vi "ZCAN_SEND.vi"(5 "CANFD_SpeedUp":u32, 6 "Data":string="11 22 33 44 55 66 77 88", 7 "ID":u32=18 format="0x%08x", 8 "error IO":errorcluster, 9 "agreement":T1, 10 "frame type":T2, 11 "can_index_handle":u32) -> (0 "error out":errorcluster)   [LabVIEW 2020, in "zlgcan.lvlib"]
uses:
  zlgcan.lvlib
  data_type/frame type.ctl
  data_type/Agreement.ctl
  data_type/ZCAN_TransmitFD_Data.ctl
  data_type/ZCAN_Transmit_Data.ctl
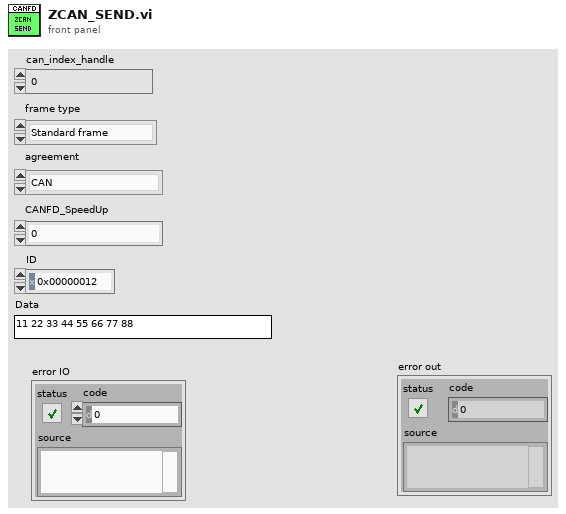
[diagram p1: front panel]
types:
  T1 = typedef "zlgcan.lvlib/Agreement.ctl" = enum16{"CAN", "CANFD"}
  T2 = typedef "zlgcan.lvlib/frame type.ctl" = enum32{"Standard frame", "Extended frame"}
  T3 = typedef "zlgcan.lvlib/ZCAN_TransmitFD_Data.ctl" = cluster{"帧类型":u32, "帧格式":u32, "ID":u32, "数据长度":u8, "CANFD加速？":u8, "DATA":cluster{"CAN数据[0]":u8, "CAN数据[1]":u8, "CAN数据[2]":u8, "CAN数据[3]":u8, "CAN数据[4]":u8, "CAN数据[5]":u8, "CAN数据[6]":u8, "CAN数据[7]":u8, "CAN数据[8]":u8, "CAN数据[9]":u8, "CAN数据[10]":u8, "CAN数据[11] ":u8, "CAN数据[12] ":u8, "CAN数据[13] ":u8, "CAN数据[14] ":u8, "CAN数据[15] ":u8, "CAN数据[16]":u8, "CAN数据[17]":u8, "CAN数据[18]":u8, "CAN数据[19]":u8, "CAN数据[20]":u8, "CAN数据[21]":u8, "CAN数据[22]":u8, "CAN数据[23]":u8, "CAN数据[24] ":u8, "CAN数据[25]":u8, "CAN数据[26]":u8, "CAN数据[27]":u8, "CAN数据[28]":u8, "CAN数据[29]":u8, "CAN数据[30]":u8, "CAN数据[31]":u8, "CAN数据[32]":u8, "CAN数据[33]":u8, "CAN数据[34]":u8, "CAN数据[35]":u8, "CAN数据[36]":u8, "CAN数据[37]":u8, "CAN数据[38]":u8, "CAN数据[39]":u8, "CAN数据[40]":u8, "CAN数据[41]":u8, "CAN数据[42]":u8, "CAN数据[43]":u8, "CAN数据[44]":u8, "CAN数据[45]":u8, "CAN数据[46]":u8, "CAN数据[47]":u8, "CAN数据[48]":u8, "CAN数据[49]":u8, "CAN数据[50]":u8, "CAN数据[51]":u8, "CAN数据[52]":u8, "CAN数据[53]":u8, "CAN数据[54]":u8, "CAN数据[55]":u8, "CAN数据[56]":u8, "CAN数据[57]":u8, "CAN数据[58]":u8, "CAN数据[59]":u8, "CAN数据[60]":u8, "CAN数据[61]":u8, "CAN数据[62]":u8, "CAN数据[63]":u8}, "发送方式":u32}
  T4 = typedef "zlgcan.lvlib/ZCAN_Transmit_Data.ctl" = cluster{"帧类型":u32, "帧格式":u32, "ID":u32, "数据长度":u8, "DATA":cluster{"CAN数据[0]":u8, "CAN数据[1]":u8, "CAN数据[2]":u8, "CAN数据[3]":u8, "CAN数据[4]":u8, "CAN数据[5]":u8, "CAN数据[6]":u8, "CAN数据[7]":u8}, "发送方式":u32}
  T5 = cluster{"[0]":u32, "[1]":u32, "[2]":u32, "[3]":u32, "[4]":u32, "[5]":u32, "[6]":u32, "[7]":u32, "[8]":u32, "[9]":u32, "[10]":u32, "[11]":u32, "[12]":u32, "[13]":u32, "[14]":u32, "[15]":u32, "[16]":u32, "[17]":u32, "[18]":u32, "[19]":u32, "[20]":u32, "[21]":u32, "[22]":u32, "[23]":u32, "[24]":u32, "[25]":u32, "[26]":u32, "[27]":u32, "[28]":u32, "[29]":u32, "[30]":u32, "[31]":u32, "[32]":u32, "[33]":u32, "[34]":u32, "[35]":u32, "[36]":u32, "[37]":u32, "[38]":u32, "[39]":u32, "[40]":u32, "[41]":u32, "[42]":u32, "[43]":u32, "[44]":u32, "[45]":u32, "[46]":u32, "[47]":u32, "[48]":u32, "[49]":u32, "[50]":u32, "[51]":u32, "[52]":u32, "[53]":u32, "[54]":u32, "[55]":u32, "[56]":u32, "[57]":u32, "[58]":u32, "[59]":u32, "[60]":u32, "[61]":u32, "[62]":u32, "[63]":u32}
  T6 = cluster{"[0]":u32, "[1]":u32, "[2]":u32, "[3]":u32, "[4]":u32, "[5]":u32, "[6]":u32, "[7]":u32}
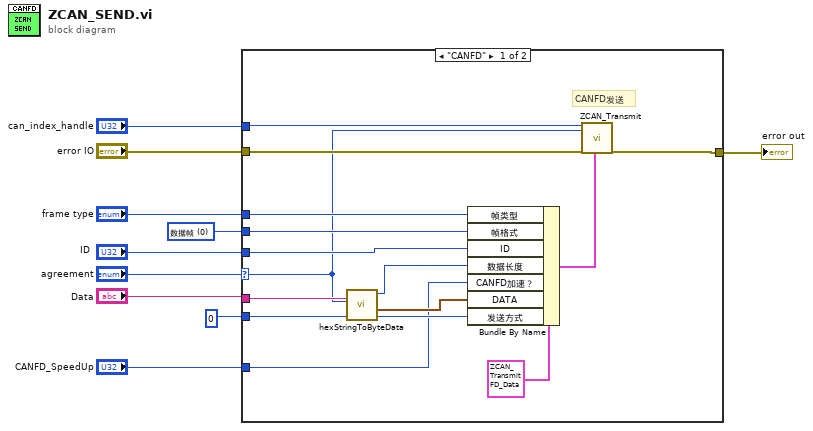
[diagram p0: block diagram]
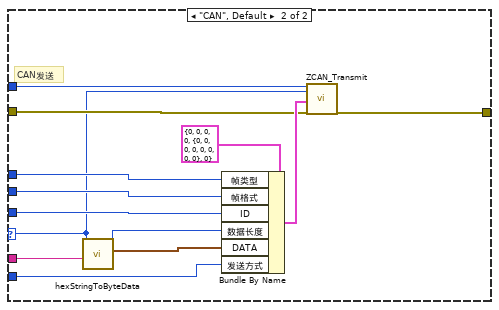
[diagram p2: hidden frame]
diagram:
  w8 = u32 0 items=["数据帧", "远程帧"] ("帧格式")
  n1 = case shown="\"CANFD\"" "agreement" {
    selector: "agreement" -> [w13 w26]
    tunnel: "frame type" -> [w23 w36]
    tunnel: w8 -> [w22 w35]
    tunnel: "ID" -> [w21 w34]
    tunnel: u32 0 ("Send Type") -> [w20 w32]
    tunnel: "Data" -> [w18 w30]
    tunnel: "error IO" -> [w16 w28]
    tunnel: "can_index_handle" -> [w14 w27]
    tunnel: [w12 w25] -> w3
    tunnel: "CANFD_SpeedUp" -> [w11 _]
    frame "CANFD" {
      # "CANFD发送"
      n2 = call "hexStringToByteData.vi"("数据输入"=w18, "协议"=w13) -> ("CANFD_data"=w19:T5, "字节数"=w17:i32)  [unwired: 7 in, 1 out]
      n3 = Bundle By Name(cluster=T3 {"帧类型"=0, "帧格式"=0, "ID"=0, "数据长度"=0, "CANFD加速？"=0, "DATA"={"CAN数据[0]"=0, "CAN数据[1]"=0, "CAN数据[2]"=0, "CAN数据[3]"=0, "CAN数据[4]"=0, "CAN数据[5]"=0, "CAN数据[6]"=0, "CAN数据[7]"=0, "CAN数据[8]"=0, "CAN数据[9]"=0, "CAN数据[10]"=0, "CAN数据[11] "=0, "CAN数据[12] "=0, "CAN数据[13] "=0, "CAN数据[14] "=0, "CAN数据[15] "=0, "CAN数据[16]"=0, "CAN数据[17]"=0, "CAN数据[18]"=0, "CAN数据[19]"=0, "CAN数据[20]"=0, "CAN数据[21]"=0, "CAN数据[22]"=0, "CAN数据[23]"=0, "CAN数据[24] "=0, "CAN数据[25]"=0, "CAN数据[26]"=0, "CAN数据[27]"=0, "CAN数据[28]"=0, "CAN数据[29]"=0, "CAN数据[30]"=0, "CAN数据[31]"=0, "CAN数据[32]"=0, "CAN数据[33]"=0, "CAN数据[34]"=0, "CAN数据[35]"=0, "CAN数据[36]"=0, "CAN数据[37]"=0, "CAN数据[38]"=0, "CAN数据[39]"=0, "CAN数据[40]"=0, "CAN数据[41]"=0, "CAN数据[42]"=0, "CAN数据[43]"=0, "CAN数据[44]"=0, "CAN数据[45]"=0, "CAN数据[46]"=0, "CAN数据[47]"=0, "CAN数据[48]"=0, "CAN数据[49]"=0, "CAN数据[50]"=0, "CAN数据[51]"=0, "CAN数据[52]"=0, "CAN数据[53]"=0, "CAN数据[54]"=0, "CAN数据[55]"=0, "CAN数据[56]"=0, "CAN数据[57]"=0, "CAN数据[58]"=0, "CAN数据[59]"=0, "CAN数据[60]"=0, "CAN数据[61]"=0, "CAN数据[62]"=0, "CAN数据[63]"=0}, "发送方式"=0} ("ZCAN_TransmitFD_Data"), "帧类型"=w23, "帧格式"=w22, "ID"=w21, "数据长度"=w17, "CANFD加速？"=w11, "DATA"=w19, "发送方式"=w20) -> (w15:T3)
      n4 = call "ZCAN_Transmit.vi"("can_index_handle"=w14, "协议"=w13, "error in (no error)"=w16, "ZCAN_TransmitFD_Data"=w15) -> ("error out"=w12:errorcluster)  [unwired: 15 in]
    }
    frame "CAN", Default {
      # "CAN发送"
      n5 = call "hexStringToByteData.vi"("数据输入"=w30, "协议"=w26) -> ("CAN_data"=w33:T6, "字节数"=w31:i32)  [unwired: 7 in, 1 out]
      n6 = Bundle By Name(cluster=T4 {"帧类型"=0, "帧格式"=0, "ID"=0, "数据长度"=0, "DATA"={"CAN数据[0]"=0, "CAN数据[1]"=0, "CAN数据[2]"=0, "CAN数据[3]"=0, "CAN数据[4]"=0, "CAN数据[5]"=0, "CAN数据[6]"=0, "CAN数据[7]"=0}, "发送方式"=0} ("ZCAN_Transmit_Data"), "帧类型"=w36, "帧格式"=w35, "ID"=w34, "数据长度"=w31, "DATA"=w33, "发送方式"=w32) -> (w29:T4)
      n7 = call "ZCAN_Transmit.vi"("can_index_handle"=w27, "协议"=w26, "ZCAN_Transmit_Data"=w29, "error in (no error)"=w28) -> ("error out"=w25:errorcluster)  [unwired: 15 in]
    }
  }
  "error out" <- w3
